vi "Write State.vi"(8 "error in (no error)":errorcluster, 10 "State":T1, 11 "Expansion in":refnum<class "Expansion.lvclass">) -> (0 "error out":errorcluster, 3 "Expansion out":refnum<class "Expansion.lvclass">)   [LabVIEW 2017, in "Expansion.lvclass"]
uses:
  Expansion.lvclass
  Type Defs/Expansion State.ctl
  Expansion.lvclass/Expansion.ctl
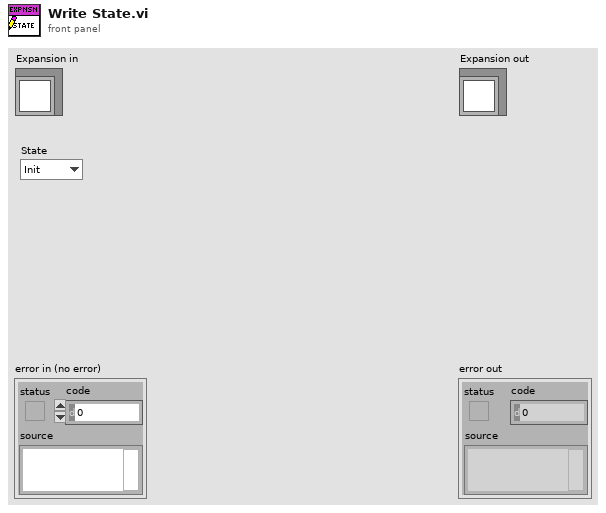
[diagram p1: front panel]
types:
  T1 = typedef "Expansion.lvclass/Expansion State.ctl" = enum16{"Init", "Go", "Move from Load to Heating", "Stop Motor", "Operate Cylinders", "Wait and Monitor", "Move from Heating to Unload", "Unload", "Move from Unload to Heating", "Move from Heating to Load", "Complete Process", "Stop", "Idle", "Error", "Shutdown"}
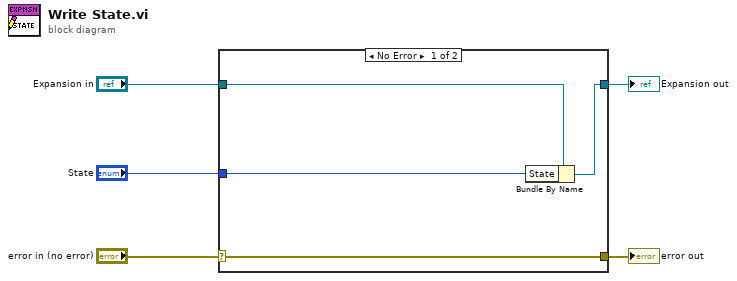
[diagram p0: block diagram]
diagram:
  n1 = case shown="No Error" "error in (no error)" {
    selector: "error in (no error)" -> [w9 w10]
    tunnel: [w9 w10] -> w4
    tunnel: [w7 w11] -> w2
    tunnel: "Expansion in" -> [w8 w11]
    tunnel: "State" -> [w6 _]
    frame No Error {
      n2 = Bundle By Name(cluster=w8, "State"=w6) -> (w7:refnum<class "Expansion.lvclass">)
    }
    frame Error {
    }
  }
  "error out" <- w4
  "Expansion out" <- w2
